vi "Check Distributed Mngr Online Status.vi"(8 "error in (no error)":errorcluster, 11 "Local Error Manager in":refnum<class "Local Error Manager.lvclass">) -> (0 "error out":errorcluster, 2 "uService online":bool, 3 "Local Error Manager out":refnum<class "Local Error Manager.lvclass">)   [LabVIEW 2026, in "TALOS.lvlib" / "Error Manager.lvlib" / "Local Error Manager.lvclass"]
uses:
  Local Error Manager.lvclass
  C:/LabVIEW Code/TALOS/talos/Father of all uServices/Father of all uServices/Father of all uServices.lvclass
  Father of all uServices/Father of all uServices/Father of all uServices.lvclass
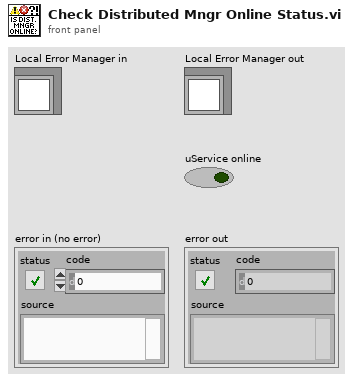
[diagram p1: front panel]
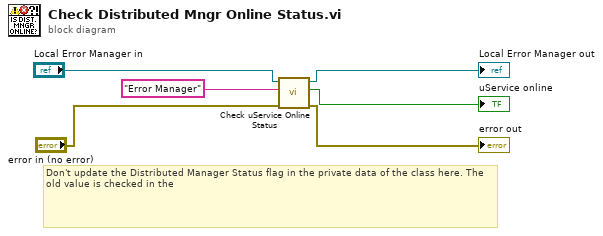
[diagram p0: block diagram]
diagram:
  # "Don't update the Distributed Manager Status flag in the private data of the class here. The old value is checked in the"
  n1 = call "Check uService Online Status.vi"("error in (no error)"="error in (no error)", "String"="Error Manager" ("uService ID"), "Father of all uServices in"="Local Error Manager in") -> ("error out"=→"error out":errorcluster, "uService online?"=→"uService online":bool, "Father of all uServices out"=→"Local Error Manager out":refnum<class "Local Error Manager.lvclass">)  [unwired: 6 in]
